vi "Format Word for CSV.vi"(8 "error in":errorcluster, 10 "data word format":T1="Hexadecimal", 11 "word":T2 {"type" format="%04x"; "activity" format="%04x"; "error" format="%04x"; "cwd1" format="%04x"; "cwd2" format="%04x"; "swd1" format="%04x"; "swd2" format="%04x"; "data" format="%04x"}) -> (0 "error out":errorcluster, 3 "string":string[](array[string]))   [LabVIEW 2020, in "Ballard MIL-STD-1553 Engine.lvlib" / "Implementation.lvlib" / "CSV Word Logger.lvclass"]
uses:
  CSV Word Logger.lvclass
  Word.ctl
  Shared/Data Word Format.ctl
  Rx Execution Unit/Rx Execution Unit.lvclass
  <instrlib>/BTI1553Lib/BTI1553LV.lvlib
  Implementation.lvlib
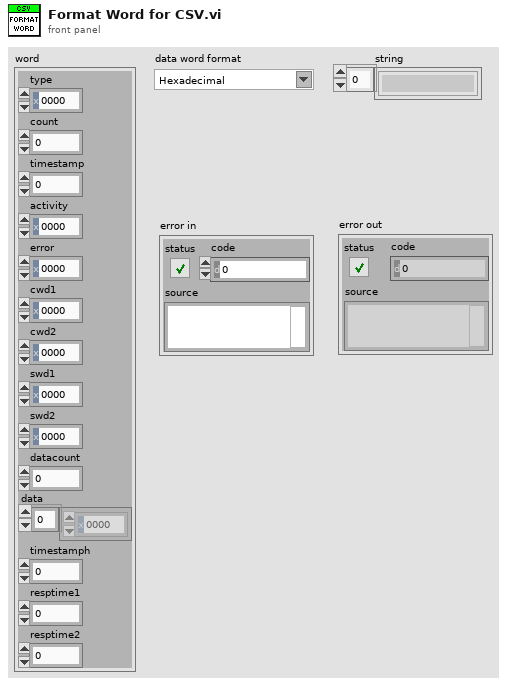
[diagram p1: front panel]
types:
  T1 = typedef "Data Word Format.ctl" = string
  T2 = typedef "Ballard MIL-STD-1553 Engine.lvlib/Implementation.lvlib/Word.ctl" = cluster{"type":u16, "count":u16, "timestamp":u32, "activity":u16, "error":u16, "cwd1":u16, "cwd2":u16, "swd1":u16, "swd2":u16, "datacount":u16, "data":u16[], "timestamph":u32, "resptime1":u16, "resptime2":u16}
  T3 = typedef "BTI1553LV.lvlib/1553 Activity Flags.ctl" = cluster{"channelnumber":i32, "transmittedcwd1":bool, "transmittedcwd2":bool, "transmittedswd1":bool, "transmittedswd2":bool, "receivedcwd1":bool, "receivedcwd2":bool, "receivedswd1":bool, "receivedswd2":bool, "transmitteddwd":bool, "receiveddwd":bool, "reserved1":i8, "reserved2":i8, "bus":u32}
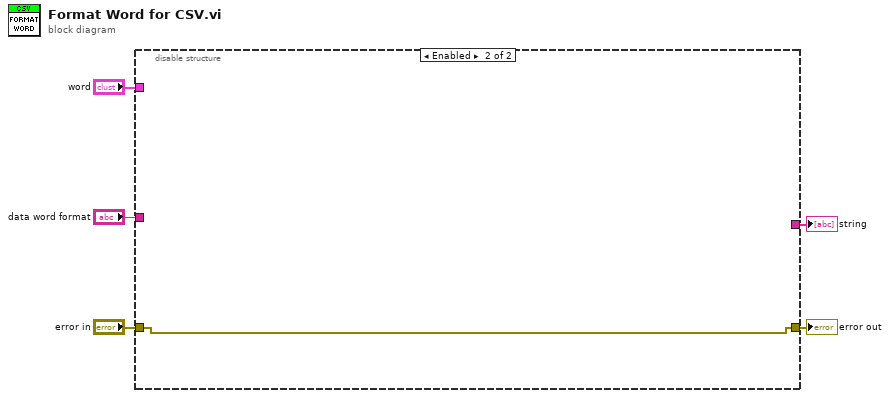
[diagram p0: block diagram]
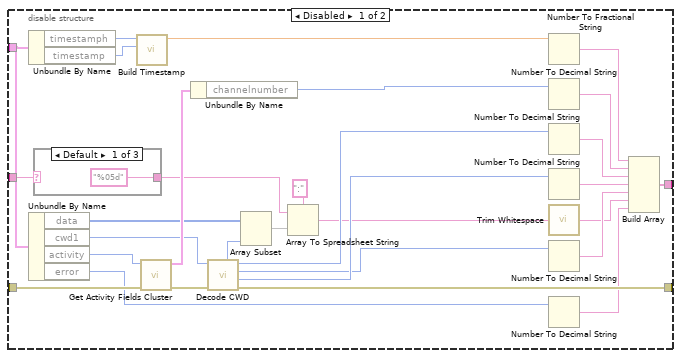
[diagram p2: hidden frame]
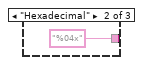
[diagram p3: hidden frame]
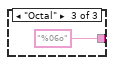
[diagram p4: hidden frame]
diagram:
  n1 = disable-structure shown="Enabled" {
    disable-tunnel: [w35 _] -> w5
    disable-tunnel: "data word format" -> [w30 _]
    disable-tunnel: "error in" -> [w25 w39]
    disable-tunnel: [w16 w39] -> w2
    disable-tunnel: "word" -> [w10 _]
    frame Disabled {
      n2 = Unbundle By Name(w10) -> ("timestamph"=w9:u32, "timestamp"=w8:u32)
      n3 = Unbundle By Name(w10) -> ("data"=w6:u16[], "cwd1"=w23:u16, "activity"=w28:u16, "error"=w7:u16)
      n4 = case shown="Default" w30 {
        tunnel: ["%05d" ("format string") "%04x" ("format string") "%06o" ("format string")] -> w18
        frame Default {
        }
        frame "Hexadecimal" {
        }
        frame "Octal" {
        }
      }
      n5 = call "Build Timestamp.vi"("timestamp low bits"=w8, "timestamp high bits"=w9) -> ("timestamp out"=w29:dbl)  [unwired: 9 in]
      n6 = call <instrlib>:"Get Activity Fields Cluster.vi"("error in (no error)"=w25, "activity"=w28) -> ("error out"=w24:errorcluster, "activity flags"=w27:T3)  [unwired: 8 in]
      n7 = Unbundle By Name(w27) -> ("channelnumber"=w26:i32)
      n8 = call <instrlib>:"Decode CWD.vi"("error in (no error)"=w24, "command word"=w23) -> ("error out"=w16:errorcluster, "subaddress out"=w21:i32, "transmit/receive bit value out"=w20:i32, "terminal address out"=w22:i32, "word count out"=w14:i32)  [unwired: 5 in]
      n9 = Array Subset(array=w6, length=w14) -> (w15:u16[])  [unwired: 1 in]
      n10 = Array To Spreadsheet String(delimiter (Tab)=":", array=w15, 3:w18) -> (spreadsheet string=w12:string)
      n11 = Number To Fractional String(number=w29) -> (F-format string=w34:string)  [unwired: 3 in]
      n12 = Number To Decimal String(number=w26) -> (decimal integer string=w31:string)  [unwired: 1 in]
      n13 = Number To Decimal String(number=w22) -> (decimal integer string=w33:string)  [unwired: 1 in]
      n14 = Number To Decimal String(number=w21) -> (decimal integer string=w32:string)  [unwired: 1 in]
      n15 = call <vilib>:"Trim Whitespace.vi"("string"=w12) -> ("trimmed string"=w11:string)  [unwired: 1 in]
      n16 = Number To Decimal String(number=w20) -> (decimal integer string=w17:string)  [unwired: 1 in]
      n17 = Number To Decimal String(number=w7) -> (decimal integer string=w13:string)  [unwired: 1 in]
      n18 = Build Array(w34, w31, w33, w32, w17, w11, w13) -> (w35:string[])
    }
    frame Enabled {
    }
  }
  "string" <- w5
  "error out" <- w2
